vi "Config_autostart.vi"(8 "error in (no error)":errorcluster, 9 "PORT":dbl=1.0 min=1.0 max=4.0 step=1.0, 10 "IOLINK MASTER NR":dbl=1.0 min=1.0 max=10.0 step=1.0, 11 "IP":string="192.168.23.100") -> (0 "error out":errorcluster)   [LabVIEW 2022 SP3]
uses:
  <vilib>/NI/Advanced HTTP Client/POST (Buffer).vi
  <vilib>/NI/Advanced HTTP Client/Session.lvclass
panel:
  # "PORT initializing"
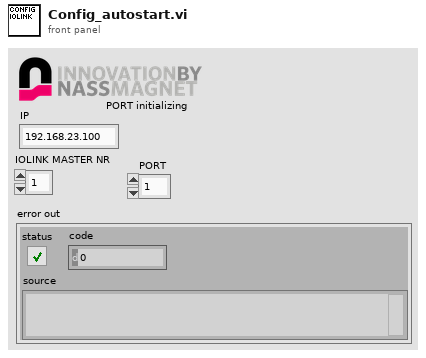
[diagram p1: front panel]
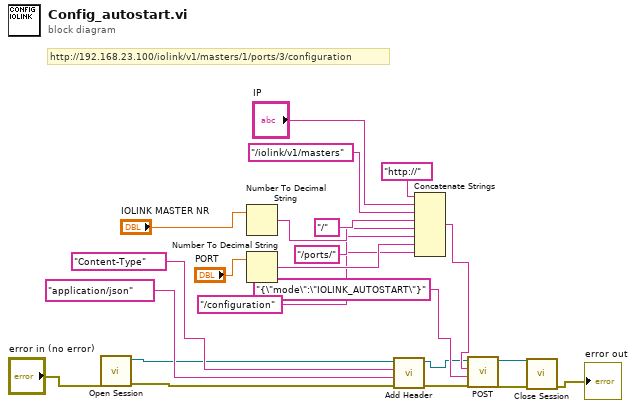
[diagram p0: block diagram]
diagram:
  # "http://192.168.23.100/iolink/v1/masters/1/ports/3/configuration"
  n1 = call <vilib>:"Open Session.vi"("error in"="error in (no error)") -> ("error out"=w5:errorcluster, "session"=w4:refnum<class "Session.lvclass">)  [unwired: 9 in]
  n2 = Number To Decimal String(number="IOLINK MASTER NR") -> (decimal integer string=w19:string)  [unwired: 1 in]
  n3 = Number To Decimal String(number="PORT") -> (decimal integer string=w15:string)  [unwired: 1 in]
  n4 = call <vilib>:"Add Header.vi"("error in"=w5, "value"="application/json" ("buffer"), "header"="Content-Type", "session in"=w4) -> ("error out"=w2:errorcluster, "session out"=w1:refnum<class "Session.lvclass">)  [unwired: 6 in]
  n5 = Concatenate Strings("http://", "IP", "/iolink/v1/masters" ("string"), "/", w19, "/ports/", w15, "/configuration") -> (w12:string)
  n6 = call-poly <vilib>:"POST.vi"("error in"=w2, "buffer"="{\"mode\":\"IOLINK_AUTOSTART\"}", "url"=w12, "session in"=w1) -> ("error out"=w6:errorcluster, "session out"=w3:refnum<class "Session.lvclass">)  [unwired: 3 in, 3 out]
  n7 = call <vilib>:"Close Session.vi"("error in"=w6, "session"=w3) -> ("error out"=→"error out":errorcluster)  [unwired: 9 in]
